vi "Enqueue Message.vi"(0 "Queue In":T1, 1 "Message":string, 2 "Message Data":variant, 3 "error in (no error)":errorcluster) -> (6 "Queue Out":T1, 9 "error out":errorcluster)   [LabVIEW 2023, in "VeriStand Console.lvlib"]
uses:
  VeriStand Console.lvlib
  TypeDefs/Message Queue.ctl
  TypeDefs/Message.ctl
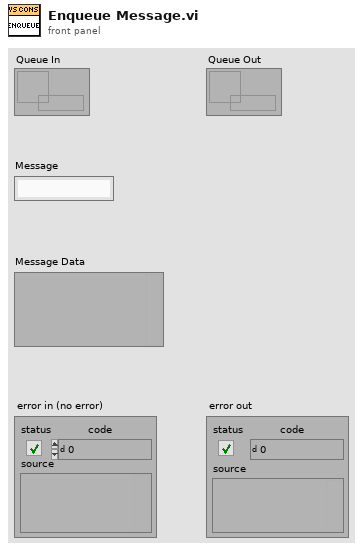
[diagram p1: front panel]
types:
  T1 = typedef "VeriStand Console.lvlib/Message Queue.ctl" = refnum<queue>
  T2 = typedef "VeriStand Console.lvlib/Message.ctl" = cluster{"Message":string, "Message Data":variant}
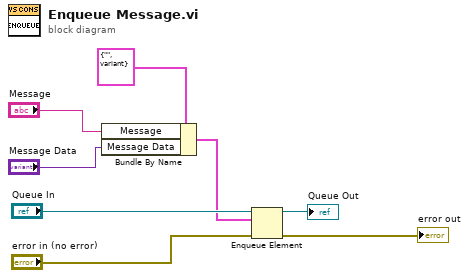
[diagram p0: block diagram]
diagram:
  n1 = Bundle By Name(cluster=T2 {"Message"="", "Message Data"=variant} ("Message"), "Message"="Message", "Message Data"="Message Data") -> (w3:T2)
  n2 = Enqueue Element(queue="Queue In", element=w3, error in (no error)="error in (no error)") -> (queue out=→"Queue Out":T1, error out=→"error out":errorcluster)  [unwired: 1 in, 1 out]
